vi "NewWafer_Dial.vi"(2 "error in (no error)":errorcluster) -> (3 "Cancelled?":bool, 4 "StartLotTraveler":T2, 6 "error out":errorcluster)   [LabVIEW 2012]
doc: "Use this template to create a dialog box with event handling."
uses:
  StartLotTraveler.ctl
  MeasurementType.ctl
panel:
  in  "Measurement Type":T1
  in  "Wafer ID":string
  in  "Cancel":bool
  in  "OK":bool
  # "Enter Wafer ID and Test Type"
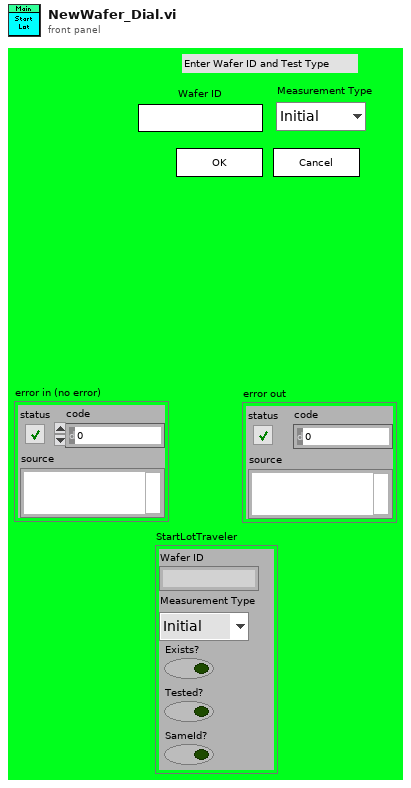
[diagram p1: front panel]
types:
  T1 = typedef "MeasurementType.ctl" = enum16{"Initial", "Final"}
  T2 = typedef "StartLotTraveler.ctl" = cluster{"Wafer ID":string, "Measurement Type":T1, "Exists?":bool, "Tested?":bool, "SameId?":bool}
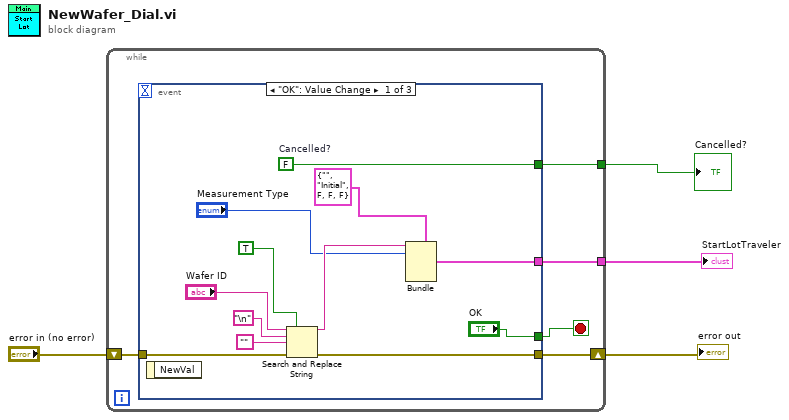
[diagram p0: block diagram]
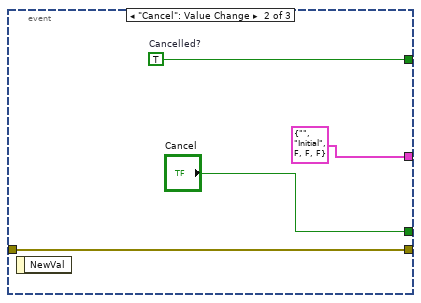
[diagram p2: hidden frame]
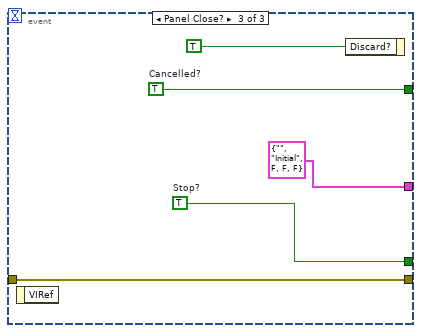
[diagram p3: hidden frame]
diagram:
  n1 = while {
    tunnel: [w8] -> w4
    shift-right: [w6] -> w3
    shift-left: "error in (no error)" -> [w7]
    tunnel: [w5] -> w1
    stop <- w9 stop-if-true
    n2 = event shown="[0] \"OK\": Value Change" {
      selector: _ -> [_ _ _]
      dyn-events: _ -> [_ _ _]
      timeout: _ -> [_ _ _]
      tunnel: ["OK" "Cancel" w29] -> w9
      tunnel: [w21 w25 w28] -> w8
      tunnel: w7 -> [w16 w23 w27]
      tunnel: [w14 w23 w27] -> w6
      tunnel: [w12 T2 {"Wafer ID"="", "Measurement Type"=enum."Initial", "Exists?"=FALSE, "Tested?"=FALSE, "SameId?"=FALSE} ("StartLotTraveler 2") T2 {"Wafer ID"="", "Measurement Type"=enum."Initial", "Exists?"=FALSE, "Tested?"=FALSE, "SameId?"=FALSE} ("StartLotTraveler 2")] -> w5
      event "OK": Value Change {
        w21 = FALSE  # Cancelled?
        n3 = event-data() -> ()  [unwired: 1 in, 1 out]
        n4 = Search and Replace String(replace all?=TRUE ("replace all? (F)"), input string="Wafer ID", search string="\n", replace string="", error in=w16) -> (result string=w13:string, error out=w14:errorcluster)  [unwired: 3 in, 2 out]
        n5 = Bundle(cluster=T2 {"Wafer ID"="", "Measurement Type"=enum."Initial", "Exists?"=FALSE, "Tested?"=FALSE, "SameId?"=FALSE} ("StartLotTraveler"), "Wafer ID"=w13, "Measurement Type"="Measurement Type") -> (w12:T2)  [unwired: 3 in]
      }
      event "Cancel": Value Change {
        w25 = TRUE  # Cancelled?
        n6 = event-data() -> ()  [unwired: 1 in, 1 out]
      }
      event Panel Close? {
        w28 = TRUE  # Cancelled?
        w29 = TRUE  # Stop?
        n7 = event-data() -> ()  [unwired: 1 in, 1 out]
        n8 = event-data("Discard?"=TRUE) -> ()  [unwired: 1 in, 1 out]
      }
    }
  }
  "Cancelled?" <- w4
  "error out" <- w3
  "StartLotTraveler" <- w1
